vi "Get Uim ICFG wrapper.vi"(8 "error in (no error)":errorcluster caption="错误输入（无错误）", 10 "dwCanNodeId":u32, 11 "dwDevIndex":u32) -> (0 "error out":errorcluster caption="错误输出", 1 "UIM_ICFG_INFO_OBJ":T1, 3 "function return":u32)   [LabVIEW 2016, in "UISimCanFunc_wrapper.lvlib"]
doc: "_declspec (dllexport) DWORD GetUimICFG_wrapper(DWORD dwDevIndex, DWORD dwCanNodeId, P_DUMMY_UIM_ICFG_INFO_OBJ pDummyICFGInfoOut);"
uses:
  <userlib>/UISimCanFunc_wrapper/UISimCanFunc_wrapper.lvlib
  <userlib>/UISimCanFunc_wrapper/ctl/UIM_ICFG_INFO_OBJ.ctl
  <userlib>/UISimCanFunc_wrapper/UISimCanFunc_wrapper.dll
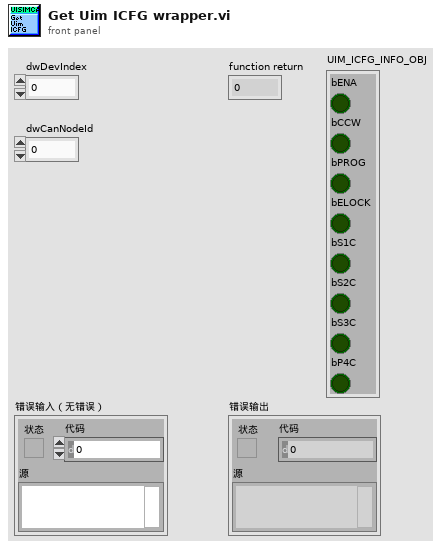
[diagram p1: front panel]
types:
  T1 = typedef "UISimCanFunc_wrapper.lvlib/UIM_ICFG_INFO_OBJ.ctl" = cluster{"bENA":bool, "bCCW":bool, "bPROG":bool, "bELOCK":bool, "bS1C":bool, "bS2C":bool, "bS3C":bool, "bP4C":bool}
  T2 = cluster{"bENA":i32, "bCCW":i32, "bPROG":i32, "bELOCK":i32, "bS1C":i32, "bS2C":i32, "bS3C":i32, "bP4C":i32}
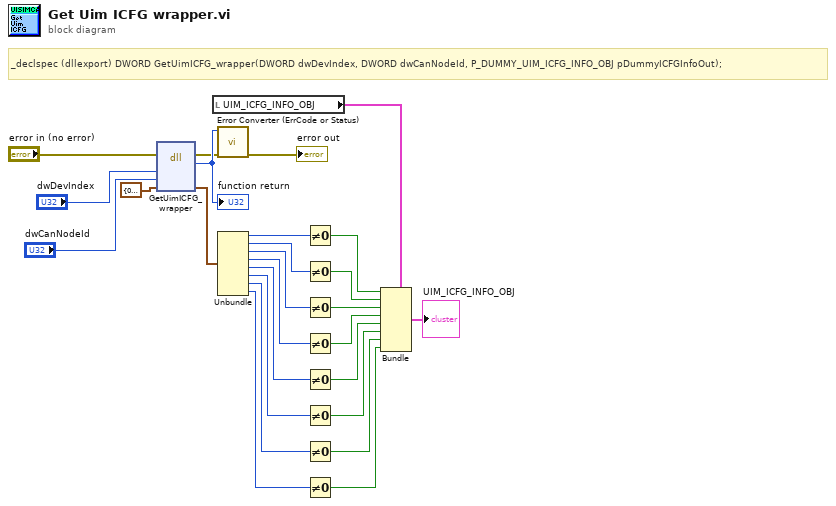
[diagram p0: block diagram]
diagram:
  # "_declspec (dllexport) DWORD GetUimICFG_wrapper(DWORD dwDevIndex, DWORD dwCanNodeId, P_DUMMY_UIM_ICFG_INFO_OBJ pDummyICFGInfoOut);"
  n1 = dll-call lib="C:/Program Files (x86)/National Instruments/LabVIEW 2016/user.lib/UISimCanFunc_wrapper/UISimCanFunc_wrapper.*" fn="GetUimICFG_wrapper"(error in="error in (no error)", "dwDevIndex"="dwDevIndex", "dwCanNodeId"="dwCanNodeId", "pDummyICFGInfoOut"=T2 {"bENA"=0, "bCCW"=0, "bPROG"=0, "bELOCK"=0, "bS1C"=0, "bS2C"=0, "bS3C"=0, "bP4C"=0}) -> (error out=w22:errorcluster, w26:u32, "pDummyICFGInfoOut"=w20:T2)  [unwired: 4 in, 1 out]
  "function return" <- w26
  n2 = local read "UIM_ICFG_INFO_OBJ"() -> (w13:T1)
  n3 = call <userlib>:"Error Converter (ErrCode or Status).vi"("error in (no error)"=w22, "error code"=w26) -> ("error out"=→"error out":errorcluster)  [unwired: 9 in]
  n4 = Unbundle(w20) -> ("bENA"=w17:i32, "bCCW"=w15:i32, "bPROG"=w12:i32, "bELOCK"=w11:i32, "bS1C"=w8:i32, "bS2C"=w7:i32, "bS3C"=w6:i32, "bP4C"=w5:i32)
  n5 = Not Equal To 0?(x=w17) -> (x != 0?=w16:bool)
  n6 = Not Equal To 0?(x=w15) -> (x != 0?=w14:bool)
  n7 = Not Equal To 0?(x=w12) -> (x != 0?=w10:bool)
  n8 = Not Equal To 0?(x=w11) -> (x != 0?=w9:bool)
  n9 = Not Equal To 0?(x=w8) -> (x != 0?=w4:bool)
  n10 = Not Equal To 0?(x=w7) -> (x != 0?=w3:bool)
  n11 = Not Equal To 0?(x=w6) -> (x != 0?=w2:bool)
  n12 = Not Equal To 0?(x=w5) -> (x != 0?=w1:bool)
  n13 = Bundle(cluster=w13, "bENA"=w16, "bCCW"=w14, "bPROG"=w10, "bELOCK"=w9, "bS1C"=w4, "bS2C"=w3, "bS3C"=w2, "bP4C"=w1) -> (→"UIM_ICFG_INFO_OBJ":T1)
